vi "ep_Broken Rotor Bars Harmonics.vi"(0 "spectra information":T1, 1 "search +/- percentage":dbl=0.025, 5 "slip":dbl[](array[numeric]), 9 "fundamental frequency [Hz]":dbl, 11 "error in (no error)":errorcluster, 12 "sinc interpolation? (F)":bool, 13 "max sideband order":i32=10) -> (4 "upper sidebands":T2(array[cluster]), 6 "lower sidebands":T2(array[cluster]), 8 "max sideband magnitude [dB]":dbl[](array[numeric]), 15 "error out":errorcluster)   [LabVIEW 2014, in "NI_EP_Motor Monitoring.lvlib"]
uses:
  <vilib>/addons/Electrical Power/Motor Monitoring/NI_EP_Motor Monitoring.lvlib
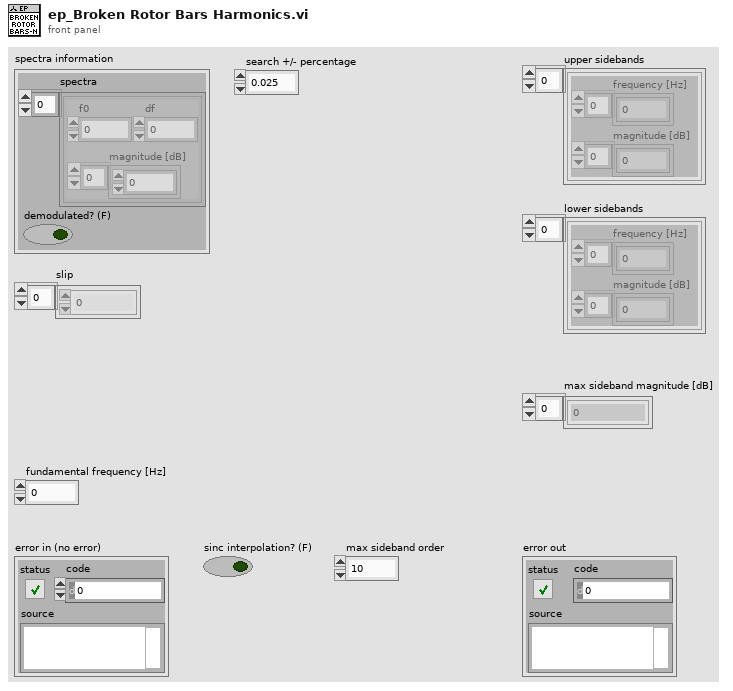
[diagram p1: front panel]
types:
  T1 = cluster{"spectra":cluster{"f0":dbl, "df":dbl, "magnitude [dB]":dbl[]}[], "demodulated? (F)":bool}
  T2 = cluster{"frequency [Hz]":dbl[], "magnitude [dB]":dbl[]}[]
  T3 = cluster{"f0":dbl, "df":dbl, "magnitude [dB]":dbl[]}[]
  T4 = cluster{"frequency [Hz]":dbl[], "magnitude [dB]":dbl[]}
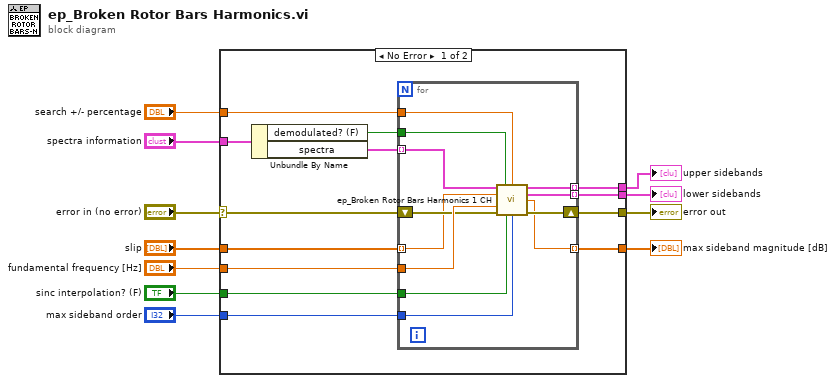
[diagram p0: block diagram]
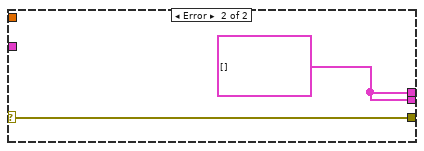
[diagram p2: hidden frame]
diagram:
  n1 = case shown="No Error" "error in (no error)" {
    selector: "error in (no error)" -> [w16 w38]
    tunnel: "slip" -> [w22 _]
    tunnel: "fundamental frequency [Hz]" -> [w21 _]
    tunnel: [w20 w37] -> w10
    tunnel: [w19 w37] -> w9
    tunnel: "spectra information" -> [w18 _]
    tunnel: [w17 w38] -> w8
    tunnel: "search +/- percentage" -> [w15 _]
    tunnel: "sinc interpolation? (F)" -> [w14 _]
    tunnel: "max sideband order" -> [w13 _]
    tunnel: [w12 _] -> w1
    frame No Error {
      n2 = Unbundle By Name(w18) -> ("demodulated? (F)"=w24:bool, "spectra"=w23:T3)
      n3 = for {
        tunnel: w23 -> [w30] mode=indexing
        tunnel: w21 -> [w35]
        shift-right: [w36] -> w17
        shift-left: w16 -> [w34]
        tunnel: w24 -> [w31]
        tunnel: [w33] -> w19 mode=indexing
        tunnel: [w32] -> w20 mode=indexing
        tunnel: w22 -> [w26] mode=indexing
        tunnel: w15 -> [w29]
        tunnel: w14 -> [w28]
        tunnel: w13 -> [w27]
        tunnel: [w25] -> w12 mode=indexing
        n4 = call <vilib>:"ep_Broken Rotor Bars Harmonics 1 CH.vi"("spectra"=w30, "demodulated? (F)"=w31, "search +/- percentage"=w29, "slip"=w26, "fundamental frequency [Hz]"=w35, "error in (no error)"=w34, "sinc interpolation? (F)"=w28, "max sideband order"=w27) -> ("upper sidebands"=w33:T4, "lower sidebands"=w32:T4, "max sideband magnitude [dB]"=w25:dbl, "error out"=w36:errorcluster)  [unwired: 4 in]
      }
    }
    frame Error {
      w37 = T2 []
    }
  }
  "lower sidebands" <- w10
  "upper sidebands" <- w9
  "error out" <- w8
  "max sideband magnitude [dB]" <- w1
